vi "YAG_Control.v5.vi"() -> ()   [LabVIEW 2018]
uses:
  YAGControl.ctl
panel:
  in  "VISA resource name":refnum<visa-resource-name>="COM1"
  in  "Cluster":T1={"Lamp mode"=TRUE, "Lamps"=FALSE, "Shutter"=FALSE, "Q-Switch"=FALSE, "Int Rep Rate  "=15.0, "Voltage "=700.0, "Temperature"=20.0, "Quit"=FALSE} {"Int Rep Rate" min=1.0 max=30.0; "Temperature" format="%#.0f"; "Voltage" min=680.0 max=950.0 step=1.0}
  in  "Send":bool
  out "Last Response":string
  in  "Other Command":string
  # "o"
  # "C"
  # "Hz"
  # "V"
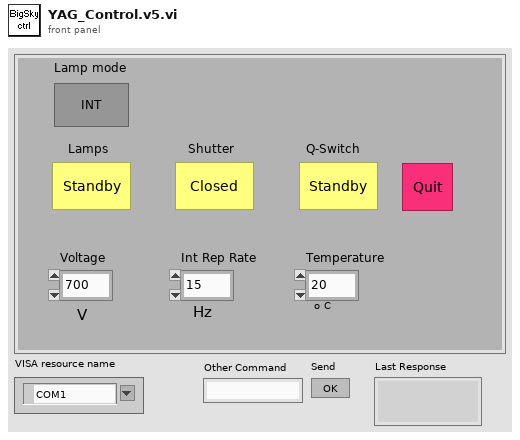
[diagram p1: front panel]
types:
  T1 = typedef "YAGControl.ctl" = cluster{"Lamp mode":bool, "Lamps":bool, "Shutter":bool, "Q-Switch":bool, "Int Rep Rate  ":dbl, "Voltage ":dbl, "Temperature":dbl, "Quit":bool}
  T2 = enum8{"Enabled", "Disabled", "Disabled and Grayed Out"}
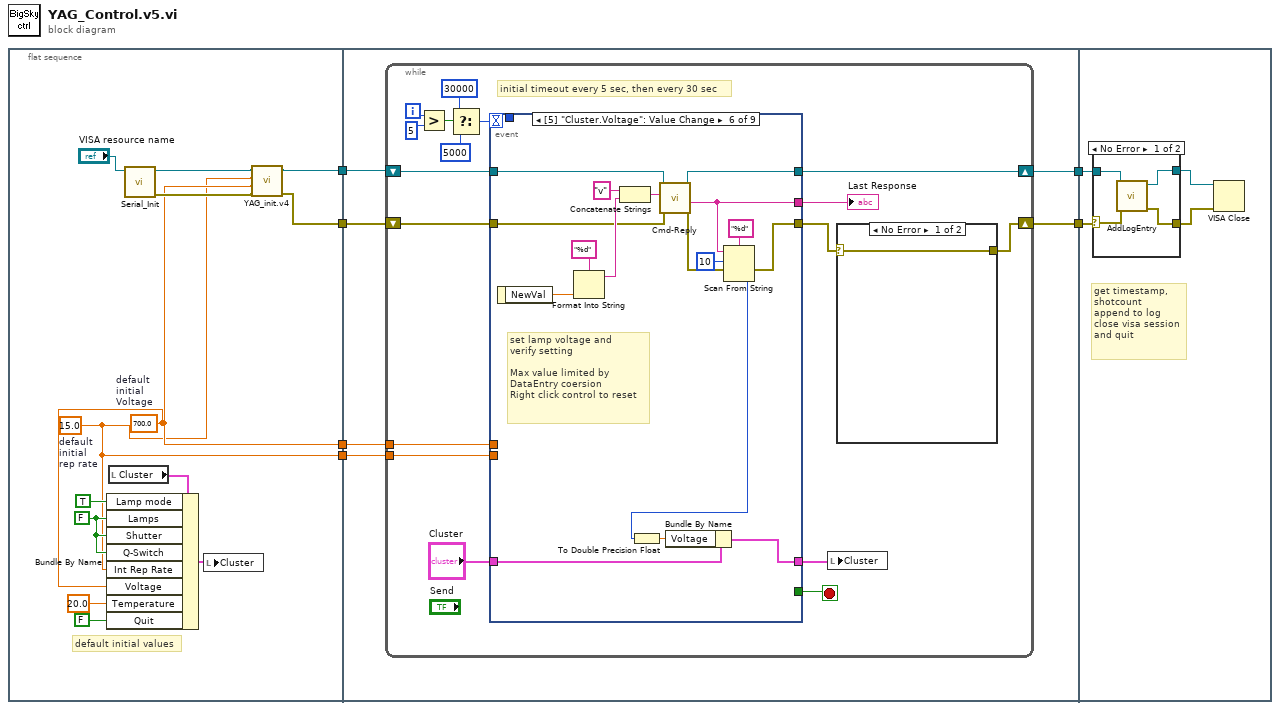
[diagram p0: block diagram]
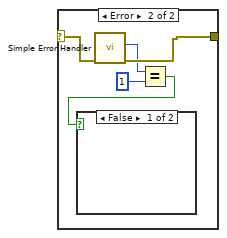
[diagram p2: hidden frame]
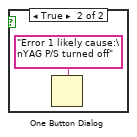
[diagram p3: hidden frame]
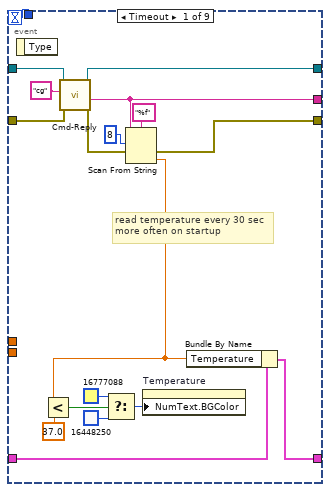
[diagram p4: hidden frame]
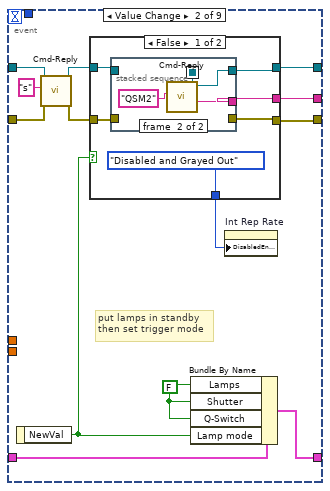
[diagram p5: hidden frame]
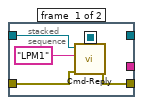
[diagram p6: hidden frame]
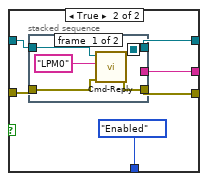
[diagram p7: hidden frame]
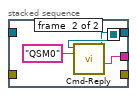
[diagram p8: hidden frame]
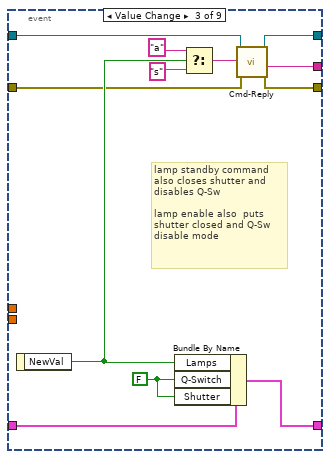
[diagram p9: hidden frame]
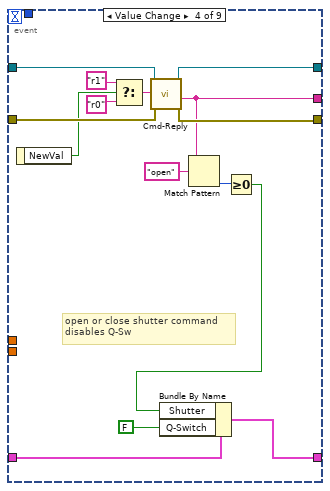
[diagram p10: hidden frame]
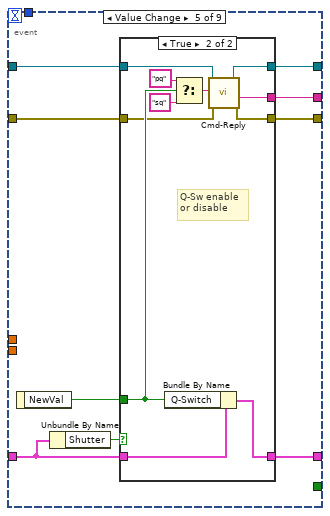
[diagram p11: hidden frame]
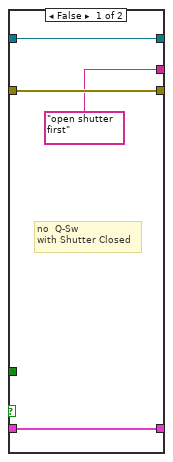
[diagram p12: hidden frame]
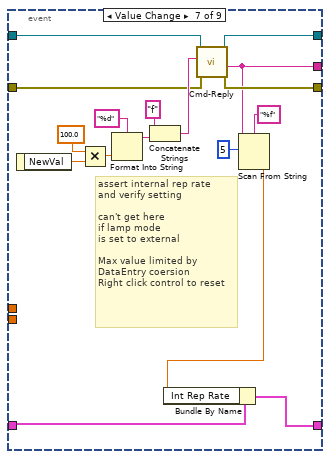
[diagram p13: hidden frame]
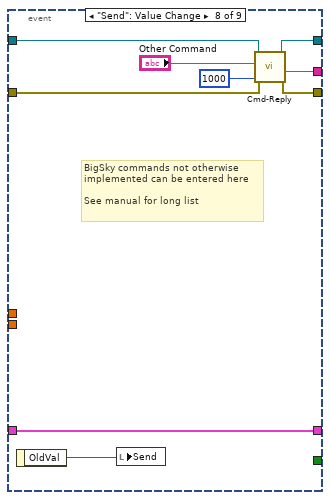
[diagram p14: hidden frame]
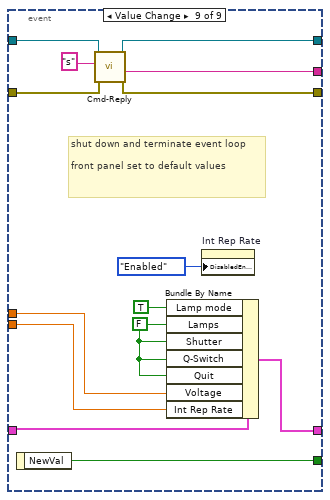
[diagram p15: hidden frame]
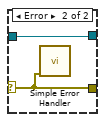
[diagram p16: hidden frame]
diagram:
  n1 = flat-sequence {
    tunnel: [w11] -> w4
    tunnel: [w10] -> w3
    tunnel: [w8] -> w2
    tunnel: [w7] -> w1
    tunnel: [w25] -> w6
    tunnel: [w24] -> w5
    tunnel: w4 -> [w23]
    tunnel: w3 -> [w22]
    tunnel: w2 -> [w21]
    tunnel: w1 -> [w20]
    tunnel: w6 -> [w219]
    tunnel: w5 -> [w222]
    frame #0 {
      w7 = 15.0  # default initial rep rate
      w8 = 700.0  # default  initial Voltage
      w18 = FALSE ("Lamp mode")
      # "default initial values"
      n2 = local read "Cluster"() -> (w13:T1)
      n3 = Bundle By Name(cluster=w13, "Lamp mode"=TRUE, "Lamps"=w18, "Shutter"=w18, "Q-Switch"=w18, "Int Rep Rate"=w7, "Voltage"=w8, "Temperature"=20.0, "Quit"=FALSE) -> (w15:T1)
      n4 = call "Serial_Init.vi"("VISA resource name"="VISA resource name") -> ("error out"=w9:errorcluster, "VISA resource name out"=w12:refnum<visa-resource-name>)  [unwired: 9 in]
      n5 = local write "Cluster"(w15) -> ()
      n6 = call "YAG_init.v4.vi"("error in (no error)"=w9, "initial V"=w8, "initial rep rate"=w7, "VISA Refnum in"=w12) -> ("error out"=w10:errorcluster, "VISA Refnum out"=w11:refnum<visa-resource-name>)  [unwired: 6 in]
    }
    frame #1 {
      n7 = while {
        shift-right: [w36] -> w24
        shift-left: w23 -> [w38]
        shift-right: [w34] -> w25
        shift-left: w22 -> [w37]
        tunnel: w21 -> [w27]
        tunnel: w20 -> [w26]
        i -> [w30]
        stop <- w42 stop-if-true
        # "initial timeout every 5 sec, then every 30 sec"
        n8 = Greater?(x=w30, y=5) -> (0:w28:bool)
        n9 = Select(t=30000, s=w28, f=5000) -> (s? t:f=w33:i32)
        n10 = event shown="[5] \"Cluster.Voltage\": Value Change" {
          selector: _ -> [_ _ _ _ _ _ _ _ _]
          dyn-events: _ -> [_ _ _ _ _ _ _ _ _]
          timeout: w33 -> [w51 _ _ _ _ _ _ _ _]
          tunnel: [_ _ _ _ _ _ _ _ w216] -> w42
          tunnel: "Cluster" -> [w67 w80 w122 w137 w144 w162 w194 w204 w218]
          tunnel: [w66 w79 w117 w136 w146 w178 w193 w204 w217] -> w39
          tunnel: [w61 w77 w116 w127 w142 w168 w183 w202 w210] -> w41
          tunnel: w38 -> [w63 w72 w112 w130 w138 w170 w185 w200 w213]
          tunnel: w37 -> [w64 w69 w113 w129 w139 w172 w184 w199 w214]
          tunnel: [w58 w73 w114 w131 w140 w164 w192 w198 w209] -> w35
          tunnel: [w62 w74 w115 w132 w141 w171 w191 w197 w211] -> w36
          tunnel: [w51 _ _ _ _ _ _ _ _] -> _
          tunnel: w27 -> [_ _ _ _ _ _ _ _ w206]
          tunnel: w26 -> [_ _ _ _ _ _ _ _ w205]
          event Timeout {
            # "read temperature every 30 sec\nmore often on startup"
            n11 = event-data() -> ()  [unwired: 1 in, 1 out]
            n12 = call "Cmd-Reply.vi"("error in (no error)"=w64, "cmd"="cg" ("write buffer"), "VISA Refnum in"=w63) -> ("error out"=w59:errorcluster, "reply"=w61:string, "VISA Refnum out"=w62:refnum<visa-resource-name>)  [unwired: 6 in]
            n13 = Scan From String(format string="%f", input string=w61, initial scan location=u32 8, error in=w59) -> (error out=w58:errorcluster, output 1=w57:dbl)  [unwired: 1 in, 2 out]
            n14 = Less?(x=w57, y=37.0) -> (x < y?=w54:bool)
            n15 = Select(t=u32 16777088 ("Color"), s=w54, f=u32 16448250 ("Color")) -> (s? t:f=w55:u32)
            n16 = property on="Temperature" class="DigNum (strict)"("NumText.BGColor"=w55) -> ()  [unwired: 2 in, 2 out]
            n17 = Bundle By Name(cluster=w67, "Temperature"=w57) -> (w66:T1)
          }
          event Value Change {
            w78 = FALSE
            # "put lamps in standby\nthen set trigger mode"
            n18 = event-data() -> ("NewVal"=w75:bool)  [unwired: 1 in]
            n19 = call "Cmd-Reply.vi"("error in (no error)"=w69, "cmd"="s" ("write buffer"), "VISA Refnum in"=w72) -> ("error out"=w68:errorcluster, "VISA Refnum out"=w71:refnum<visa-resource-name>)  [unwired: 6 in, 1 out]
            n20 = case shown="False" w75 {
              tunnel: [w81 w96] -> w77
              tunnel: [T2."Disabled and Grayed Out" ("Disabled") T2."Enabled" ("Disabled")] -> w76
              tunnel: [w85 w99] -> w74
              tunnel: [w84 w97] -> w73
              tunnel: w71 -> [w83 w100]
              tunnel: w68 -> [w82 w98]
              frame False {
                n21 = stacked-sequence {
                  seq-local: [w87 _] -> [_ w93]
                  tunnel: [_ w92] -> w85
                  tunnel: [w91 _] -> w84
                  tunnel: w83 -> [w90 _]
                  tunnel: w82 -> [w89 _]
                  tunnel: [_ w94] -> w81
                  frame #0 {
                    n22 = call "Cmd-Reply.vi"("error in (no error)"=w89, "cmd"="LPM1", "VISA Refnum in"=w90) -> ("error out"=w91:errorcluster, "VISA Refnum out"=w87:refnum<visa-resource-name>)  [unwired: 6 in, 1 out]
                  }
                  frame #1 {
                    n23 = call "Cmd-Reply.vi"("cmd"="QSM2", "VISA Refnum in"=w93) -> ("reply"=w94:string, "VISA Refnum out"=w92:refnum<visa-resource-name>)  [unwired: 7 in, 1 out]
                  }
                }
              }
              frame True {
                n24 = stacked-sequence {
                  seq-local: [w102 _] -> [_ w109]
                  tunnel: w100 -> [w105 _]
                  tunnel: [_ w108] -> w99
                  tunnel: w98 -> [w104 _]
                  tunnel: [w103 _] -> w97
                  tunnel: [_ w107] -> w96
                  frame #0 {
                    n25 = call "Cmd-Reply.vi"("error in (no error)"=w104, "cmd"="LPM0", "VISA Refnum in"=w105) -> ("error out"=w103:errorcluster, "VISA Refnum out"=w102:refnum<visa-resource-name>)  [unwired: 6 in, 1 out]
                  }
                  frame #1 {
                    n26 = call "Cmd-Reply.vi"("cmd"="QSM0", "VISA Refnum in"=w109) -> ("reply"=w107:string, "VISA Refnum out"=w108:refnum<visa-resource-name>)  [unwired: 7 in, 1 out]
                  }
                }
              }
            }
            n27 = Bundle By Name(cluster=w80, "Lamps"=w78, "Shutter"=w78, "Q-Switch"=w78, "Lamp mode"=w75) -> (w79:T1)
            n28 = property on="Int Rep Rate" class="DigNum (strict)"("DisabledEnum"=w76) -> ()  [unwired: 2 in, 2 out]
          }
          event Value Change {
            w118 = FALSE
            # "lamp standby command\nalso closes shutter and\ndisables Q-Sw\n\nlamp enable also  puts\nshutter closed and Q-Sw \ndisable mode"
            n29 = event-data() -> ("NewVal"=w119:bool)  [unwired: 1 in]
            n30 = Bundle By Name(cluster=w122, "Lamps"=w119, "Q-Switch"=w118, "Shutter"=w118) -> (w117:T1)
            n31 = Select(t="a", s=w119, f="s") -> (s? t:f=w111:string)
            n32 = call "Cmd-Reply.vi"("error in (no error)"=w113, "cmd"=w111, "VISA Refnum in"=w112) -> ("error out"=w114:errorcluster, "reply"=w116:string, "VISA Refnum out"=w115:refnum<visa-resource-name>)  [unwired: 6 in]
          }
          event Value Change {
            # "open or close shutter command\ndisables Q-Sw"
            n33 = event-data() -> ("NewVal"=w124:bool)  [unwired: 1 in]
            n34 = Select(t="r1", s=w124, f="r0") -> (s? t:f=w128:string)
            n35 = call "Cmd-Reply.vi"("error in (no error)"=w129, "cmd"=w128, "VISA Refnum in"=w130) -> ("error out"=w131:errorcluster, "reply"=w127:string, "VISA Refnum out"=w132:refnum<visa-resource-name>)  [unwired: 6 in]
            n36 = Match Pattern(string=w127, regular expression="open") -> (offset past match=w125:i32)  [unwired: 1 in, 3 out]
            n37 = Greater Or Equal To 0?(x=w125) -> (x >= 0?=w123:bool)
            n38 = Bundle By Name(cluster=w137, "Shutter"=w123, "Q-Switch"=FALSE) -> (w136:T1)
          }
          event Value Change {
            n39 = event-data() -> ("NewVal"=w145:bool)  [unwired: 1 in]
            n40 = Unbundle By Name(w144) -> ("Shutter"=w143:bool)
            n41 = case shown="True" w143 {
              tunnel: [w150 w157] -> w146
              tunnel: w145 -> [_ w158]
              tunnel: w144 -> [w150 w161]
              tunnel: ["open shutter first" w156] -> w142
              tunnel: [w149 w155] -> w141
              tunnel: [w148 w154] -> w140
              tunnel: w139 -> [w148 w153]
              tunnel: w138 -> [w149 w152]
              frame False {
                # "no  Q-Sw \nwith Shutter Closed"
              }
              frame True {
                # "Q-Sw enable\nor disable"
                n42 = Bundle By Name(cluster=w161, "Q-Switch"=w158) -> (w157:T1)
                n43 = Select(t="pq", s=w158, f="sq") -> (s? t:f=w151:string)
                n44 = call "Cmd-Reply.vi"("error in (no error)"=w153, "cmd"=w151, "VISA Refnum in"=w152) -> ("error out"=w154:errorcluster, "reply"=w156:string, "VISA Refnum out"=w155:refnum<visa-resource-name>)  [unwired: 6 in]
              }
            }
          }
          event Value Change {
            # "set lamp voltage and\nverify setting\n\nMax value limited by\nDataEntry coersion \nRight click control to reset"
            n45 = event-data() -> ("NewVal"=w176:dbl)  [unwired: 1 in]
            n46 = Format Into String(format string="%d", w176) -> (resulting string=w174:string)  [unwired: 2 in, 1 out]
            n47 = Concatenate Strings("v" ("string"), w174) -> (w175:string)
            n48 = call "Cmd-Reply.vi"("error in (no error)"=w172, "cmd"=w175, "VISA Refnum in"=w170) -> ("error out"=w165:errorcluster, "reply"=w168:string, "VISA Refnum out"=w171:refnum<visa-resource-name>)  [unwired: 6 in]
            n49 = Scan From String(format string="%d", input string=w168, initial scan location=u32 10, error in=w165) -> (error out=w164:errorcluster, output 1=w169:i32)  [unwired: 1 in, 2 out]
            n50 = To Double Precision Float(number=w169) -> (double precision float=w163:dbl)
            n51 = Bundle By Name(cluster=w162, "Voltage"=w163) -> (w178:T1)
          }
          event Value Change {
            # "assert internal rep rate\nand verify setting\n\ncan't get here  \nif lamp mode\nis set to external\n\nMax value limited by\nDataEntry coersion \nRight click control to reset"
            n52 = event-data() -> ("NewVal"=w180:dbl)  [unwired: 1 in]
            n53 = Multiply(x=100.0, y=w180) -> (x*y=w188:dbl)
            n54 = Format Into String(format string="%d", w188) -> (resulting string=w186:string)  [unwired: 2 in, 1 out]
            n55 = Concatenate Strings("f" ("string"), w186) -> (w190:string)
            n56 = call "Cmd-Reply.vi"("error in (no error)"=w184, "cmd"=w190, "VISA Refnum in"=w185) -> ("error out"=w192:errorcluster, "reply"=w183:string, "VISA Refnum out"=w191:refnum<visa-resource-name>)  [unwired: 6 in]
            n57 = Scan From String(format string="%f", input string=w183, initial scan location=u32 5) -> (output 1=w179:dbl)  [unwired: 2 in, 3 out]
            n58 = Bundle By Name(cluster=w194, "Int Rep Rate"=w179) -> (w193:T1)
          }
          event "Send": Value Change {
            # "BigSky commands not otherwise\nimplemented can be entered here\n\nSee manual for long list"
            n59 = event-data() -> ("OldVal"=w203:bool)  [unwired: 1 in]
            n60 = local write "Send"(w203) -> ()
            n61 = call "Cmd-Reply.vi"("error in (no error)"=w199, "ms to wait"=u32 1000, "cmd"="Other Command", "VISA Refnum in"=w200) -> ("error out"=w198:errorcluster, "reply"=w202:string, "VISA Refnum out"=w197:refnum<visa-resource-name>)  [unwired: 5 in]
          }
          event Value Change {
            w215 = FALSE
            # "shut down and terminate event loop\n\nfront panel set to default values"
            n62 = event-data() -> ("NewVal"=w216:bool)  [unwired: 1 in]
            n63 = call "Cmd-Reply.vi"("error in (no error)"=w214, "cmd"="s", "VISA Refnum in"=w213) -> ("error out"=w209:errorcluster, "reply"=w210:string, "VISA Refnum out"=w211:refnum<visa-resource-name>)  [unwired: 6 in]
            n64 = Bundle By Name(cluster=w218, "Lamp mode"=TRUE, "Lamps"=w215, "Shutter"=w215, "Q-Switch"=w215, "Quit"=w215, "Voltage"=w206, "Int Rep Rate"=w205) -> (w217:T1)
            n65 = property on="Int Rep Rate" class="DigNum (strict)"("DisabledEnum"=T2."Enabled" ("Disabled")) -> ()  [unwired: 2 in, 2 out]
          }
        }
        "Last Response" <- w41
        n66 = local write "Cluster"(w39) -> ()
        n67 = case shown="No Error" w35 {
          selector: w35 -> [w43 w48]
          tunnel: [w43 w47] -> w34
          frame No Error {
          }
          frame Error {
            n68 = call <vilib>:"Simple Error Handler.vi"("error in (no error)"=w48) -> ("code out"=w46:i32, "error out"=w47:errorcluster)  [unwired: 4 in, 3 out]
            n69 = Equal?(x=w46, y=1) -> (x = y?=w44:bool)
            n70 = case shown="False" w44 {
              frame False {
              }
              frame True {
                n71 = One Button Dialog(message="Error 1 likely cause:\nYAG P/S turned off") -> ()  [unwired: 1 in, 1 out]
              }
            }
          }
        }
      }
    }
    frame #2 {
      # "get timestamp,\nshotcount\nappend to log\nclose visa session\nand quit"
      n72 = case shown="No Error" w219 {
        selector: w219 -> [w223 w227]
        tunnel: w222 -> [w226 w228]
        tunnel: [w225 w227] -> w221
        tunnel: [w224 w228] -> w220
        frame No Error {
          n73 = call "AddLogEntry.vi"("error in"=w223, "VISA Refnum in"=w226) -> ("error out"=w225:errorcluster, "VISA Refnum out"=w224:refnum<visa-resource-name>)  [unwired: 8 in]
        }
        frame Error {
          n74 = call <vilib>:"Simple Error Handler.vi"("error in (no error)"=w227) -> ()  [unwired: 4 in, 5 out]
        }
      }
      n75 = VISA Close(VISA resource name=w220, error in (no error)=w221) -> ()  [unwired: 1 out]
    }
  }
